vi "load_config_v4.vi"(8 "Config Directory":path=path "D:/ParDates") -> (10 "Noff_laser":u32 step=1, 12 "USED_FILTERS":u8[](array[numeric]), 14 "USED_LEDS":bool[][](array[boolean]), 15 "NPAT":u32, 16 "EXPT":dbl, 17 "BETWEEN_SCAN":u32, 18 "Non_laser":u32=150 step=1, 19 "NSCAN":u32, 20 "Refnum VISA en sortie":refnum<visa-resource-name>="COM1", 21 "BIN":u16, 22 "Nstart_laser":u32=30 step=1, 23 "ROMODE":u32, 24 "BETWEEN_PAT":u32, 25 "STAGE_SPEED":dbl, 26 "XYPOS":T1)   [LabVIEW 2013]
uses:
  <vilib>/Analysis/Matrix/Datatypes/RealMatrix.ctl
  <vilib>/Analysis/Matrix/NI_Matrix.lvlib
panel:
  out "MIN_SCAN_DUR":dbl
  out "Nstart_fluidics":u32=30 step=1
  out "Non_fluidics":u32=150 step=1
  out "Noff_fluidics":u32 step=1
  out "shoot_duration":dbl
  out "shoot_at_SCAN":u32
  out "useFLUIDICS":bool
  out "isSINGLEshoot":bool
  out "useLASER":bool
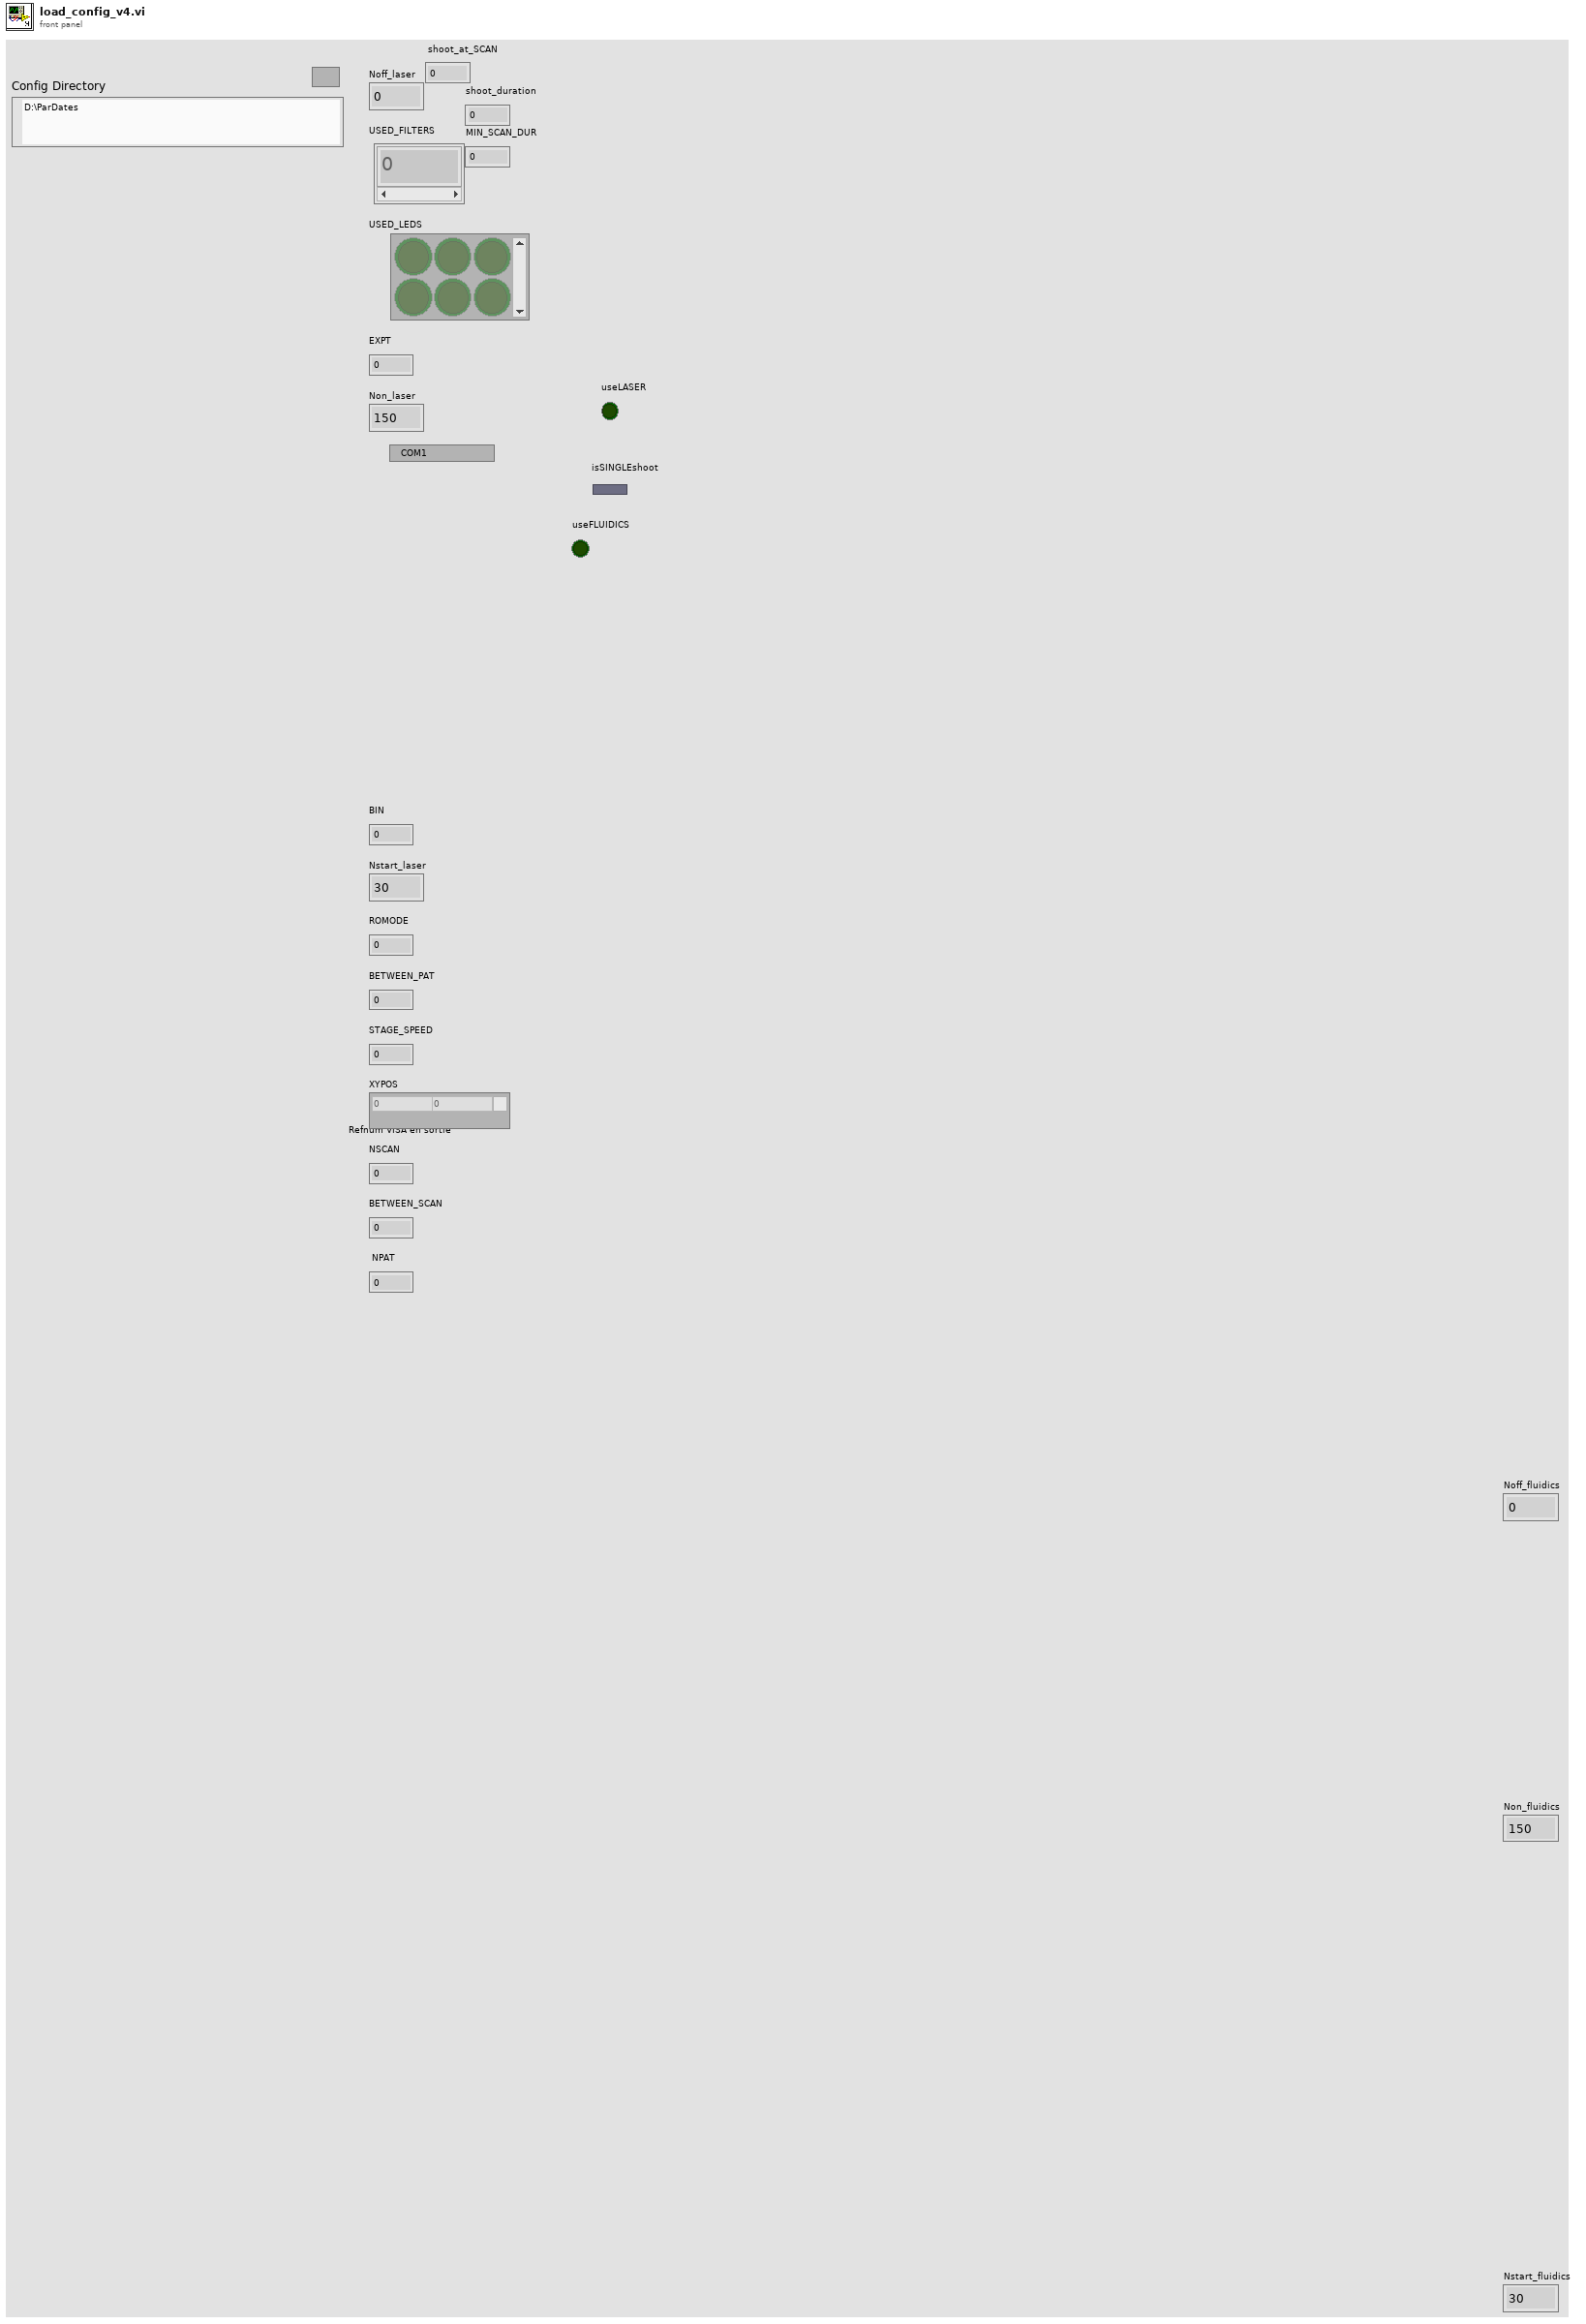
[diagram p1: front panel]
types:
  T1 = typedef "NI_Matrix.lvlib/RealMatrix.ctl" = dbl[][]
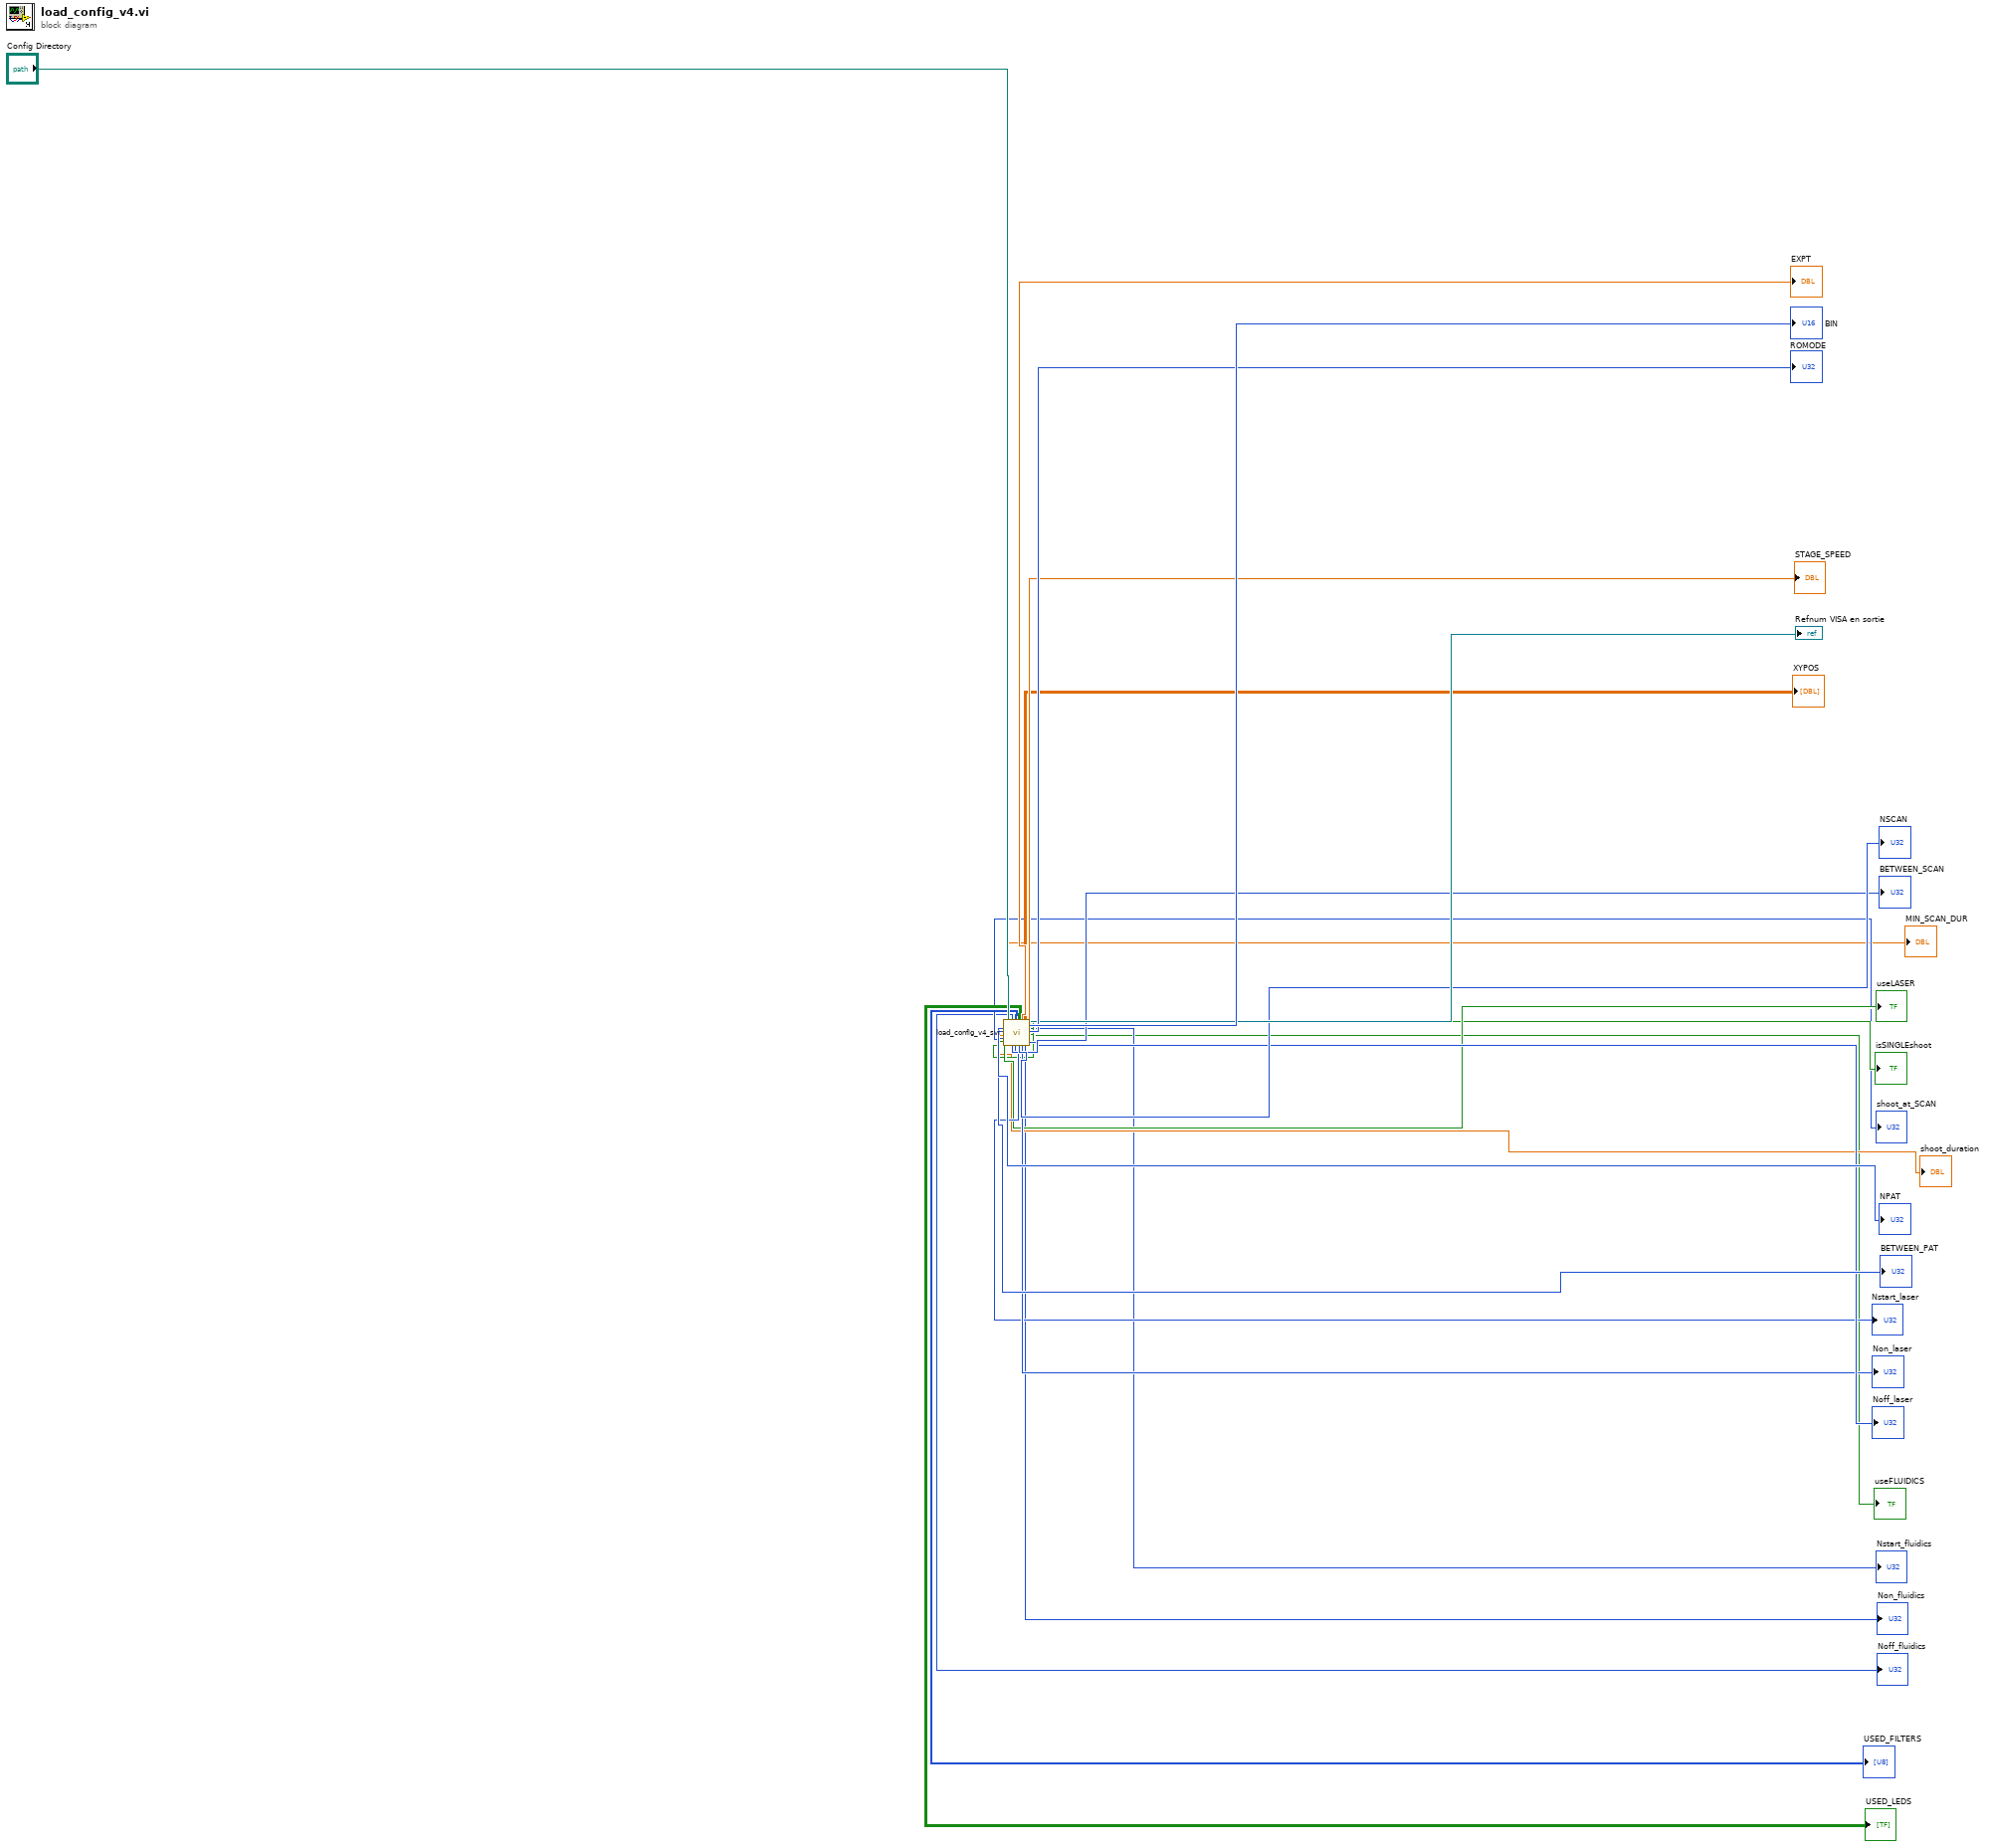
[diagram p0: block diagram]
diagram:
  n1 = call "load_config_v4_svi.vi"("Config Directory"="Config Directory") -> ("Numérique 10"=→"BETWEEN_PAT":u32, "Numérique 11"=→"NPAT":u32, "Numérique 5"=→"shoot_duration":dbl, "Numérique 6"=→"shoot_at_SCAN":u32, "Booléen 2"=→"isSINGLEshoot":bool, "Booléen 3"=→"useLASER":bool, "Numérique"=→"MIN_SCAN_DUR":dbl, "Numérique 2"=→"Noff_fluidics":u32, "Numérique 12"=→"BETWEEN_SCAN":u32, "USED_FILTERS 2"=→"USED_FILTERS":u8[], "Numérique 7"=→"Nstart_laser":u32, "USED_LEDS 2"=→"USED_LEDS":bool[][], "Numérique 13"=→"NSCAN":u32, "Numérique 17"=→"EXPT":dbl, "Numérique 8"=→"Non_laser":u32, "Numérique 3"=→"Non_fluidics":u32, "XYPOS 2"=→"XYPOS":T1, "Refnum VISA en sortie"=→"Refnum VISA en sortie":refnum<visa-resource-name>, "Numérique 16"=→"BIN":u16, "Numérique 4"=→"Nstart_fluidics":u32, "Numérique 15"=→"ROMODE":u32, "Booléen"=→"useFLUIDICS":bool, "Numérique 14"=→"STAGE_SPEED":dbl, "Numérique 9"=→"Noff_laser":u32)  [unwired: 3 in]
